vi "Reshape.vi"(6 "Numeric":i32, 9 "EEG_Channel_Num":i32, 10 "all rows":dbl[][](array[numeric]), 11 "Numeric 2":dbl) -> (3 "Array":dbl[][](array[numeric]))   [LabVIEW 2014]
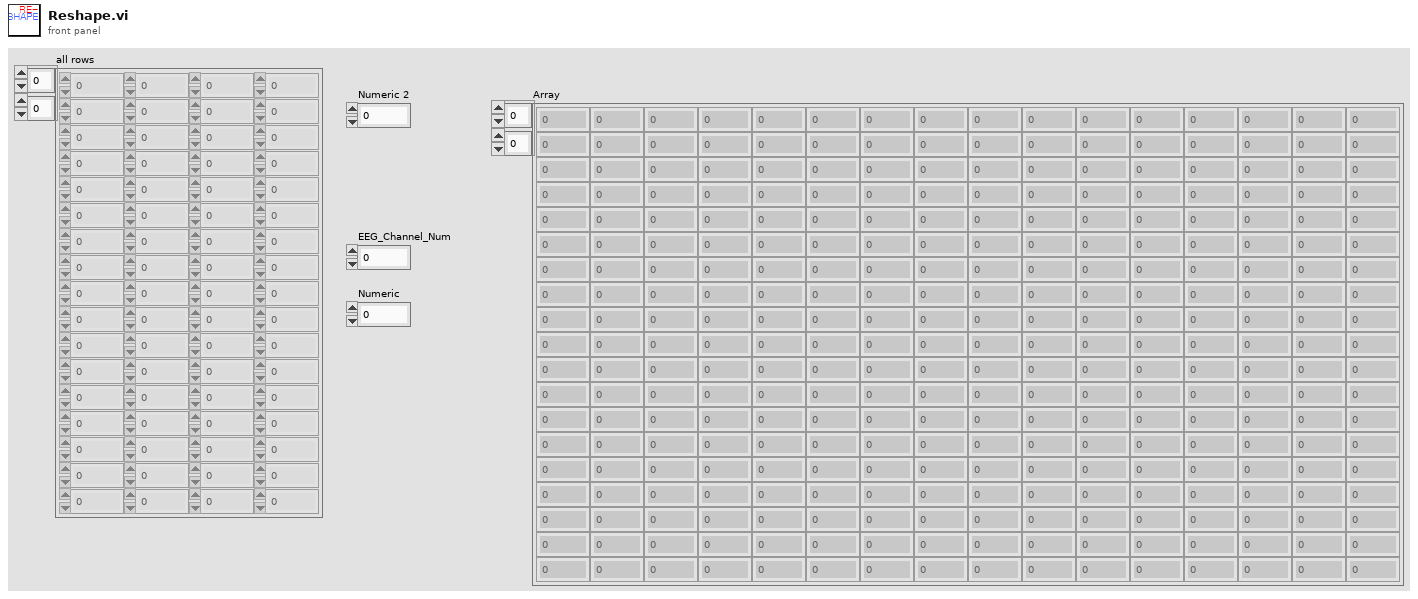
[diagram p1: front panel]
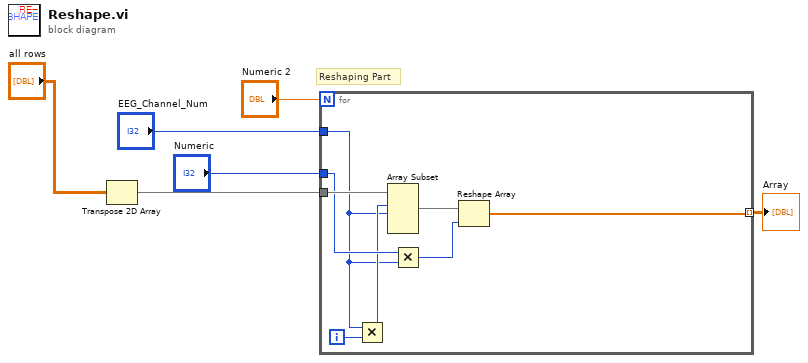
[diagram p0: block diagram]
diagram:
  # "Reshaping Part"
  n1 = Transpose 2D Array(2D array="all rows") -> (transposed array=w1:dbl[][])
  n2 = for {
    N: "Numeric 2" -> [_]
    tunnel: "EEG_Channel_Num" -> [w7]
    tunnel: w1 -> [w14]
    tunnel: "Numeric" -> [w10]
    tunnel: [w11] -> w6 mode=indexing
    i -> [w13]
    n3 = Multiply(x=w7, y=w13) -> (x*y=w8:i32)
    n4 = Array Subset(array=w14, index (row)=w8, length (row)=w7) -> (w12:dbl[][])  [unwired: 2 in]
    n5 = Multiply(x=w10, y=w7) -> (x*y=w9:i32)
    n6 = Reshape Array(w12, w9) -> (w11:dbl[])
  }
  "Array" <- w6
